vi "Get Reduced Pressure.vi"(6 "Etalon":enum16{"absolute", "related"}(ring), 8 "error in (no error)":errorcluster, 9 "Pressure unit":enum16{"bar", "MPa"}(ring), 11 "Sensor General Class in":refnum<class "Sensor General Class.lvclass">) -> (0 "error out":errorcluster, 2 "Reduced Pressure":sgl, 3 "Sensor General Class out":refnum<class "Sensor General Class.lvclass">)   [LabVIEW 2020, in "Sensor General Class.lvclass"]
uses:
  Sensor General Class.lvclass
  Data Enum.ctl
  Sensor General Class.lvclass/Sensor General Class.ctl
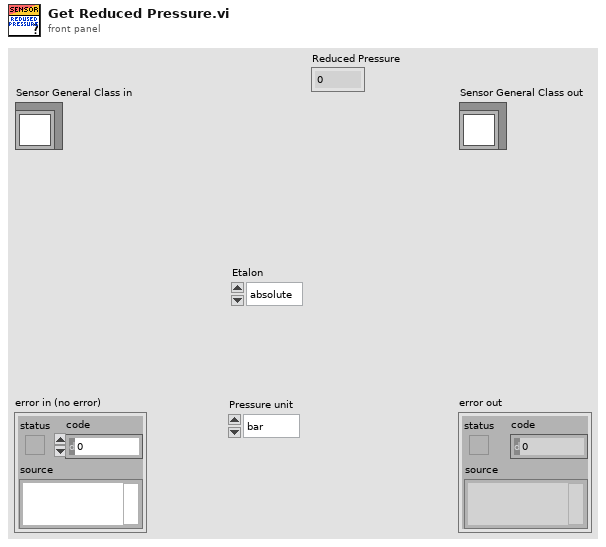
[diagram p1: front panel]
types:
  T1 = typedef "Sensor General Class.lvclass/Data Enum.ctl" = enum16{"p_bar", "p_MPa", "p_Pa", "p_kPa", "p_psi", "p_H/cm^2", "t_C", "t_K", "t_F", "rho_g/l", "rho_kg/m^3", "p20_bar", "related p20_bar", "p20_MPa", "related p20_MPa", "Tf_SF6", "Td_sf6", "tank Tf_SF6", "tank Td_SF6", "Tf_N2", "Td_N2", "tank Tf_N2", "tank Td_N2", "ppm_v SF6", "ppm_w SF6", "ppm_v N2", "ppm_w N2", "rH", "errors"}
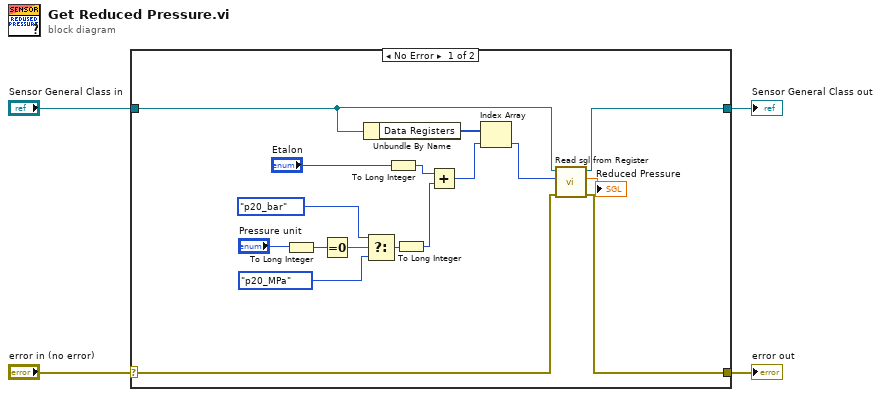
[diagram p0: block diagram]
diagram:
  n1 = case shown="No Error" "error in (no error)" {
    selector: "error in (no error)" -> [w7 w23]
    tunnel: [w6 w23] -> w3
    tunnel: [w15 w22] -> w1
    tunnel: "Sensor General Class in" -> [w16 w22]
    frame No Error {
      n2 = To Long Integer(number="Pressure unit") -> (32bit integer=w14:i32)
      n3 = Equal To 0?(x=w14) -> (x = 0?=w13:bool)
      n4 = Unbundle By Name(w16) -> ("Data Registers"=w19:u16[])
      n5 = Select(t=Data_Enum."p20_bar" ("Data Enum"), s=w13, f=Data_Enum."p20_MPa" ("Data Enum")) -> (s? t:f=w10:T1)
      n6 = To Long Integer(number="Etalon") -> (32bit integer=w20:i32)
      n7 = To Long Integer(number=w10) -> (32bit integer=w9:i32)
      n8 = Add(x=w20, y=w9) -> (x+y=w18:i32)
      n9 = Index Array(array=w19, index=w18) -> (element=w17:u16)
      n10 = call-dynamic "Read sgl from Register.vi"("error in (no error)"=w7, "Start Register"=w17, "Sensor General Class in"=w16) -> ("error out"=w6:errorcluster, "Data"=→"Reduced Pressure":sgl, "Sensor General Class out"=w15:refnum<class "Sensor General Class.lvclass">)  [unwired: 6 in]
    }
    frame Error {
    }
  }
  "error out" <- w3
  "Sensor General Class out" <- w1
